vi "LOX Crossover Template.vi"(6 "Array Size":i32=9, 8 "Index 2":i32=5, 9 "Index 1":i32=3, 10 "Schedule 2":u16[](array[numeric])=[3, 7, 8, 1, 4, 9, 2, 5, 6], 11 "Schedule 1":u16[](array[numeric])=[1, 3, 2, 6, 4, 5, 9, 7, 8]) -> (3 "Child":u16[](array[numeric]))   [LabVIEW 2013, in "GA.lvclass"]
uses:
  GA.lvclass
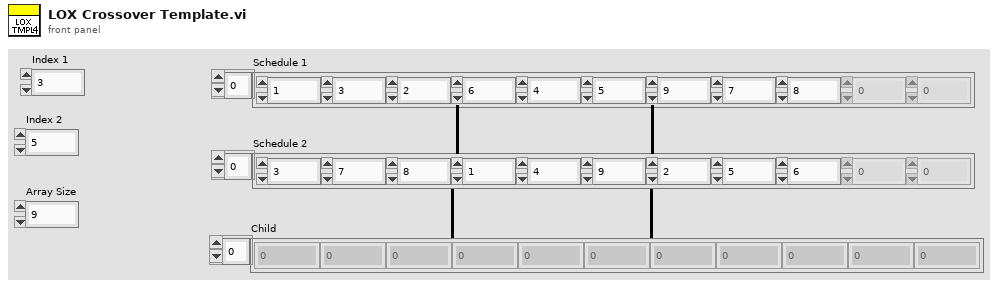
[diagram p1: front panel]
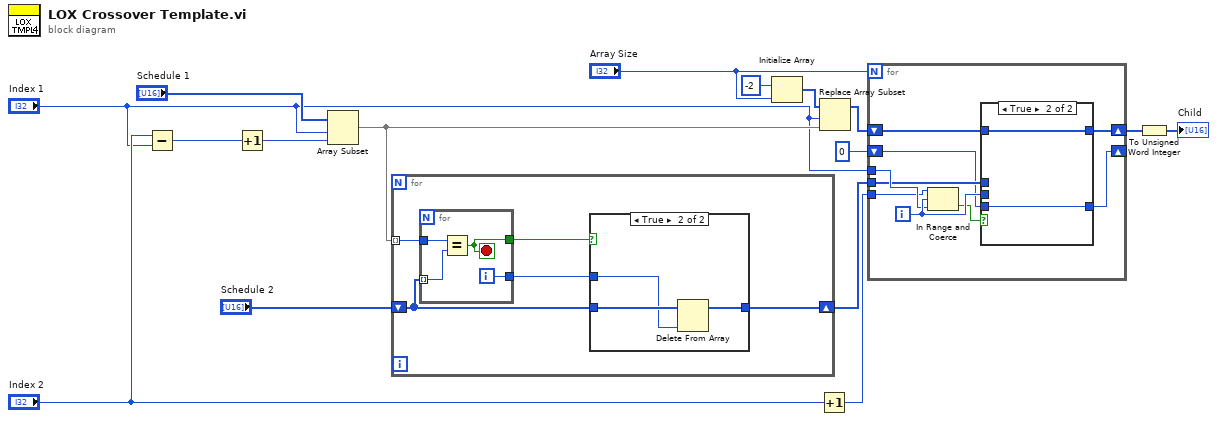
[diagram p0: block diagram]
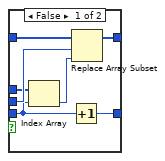
[diagram p2: hidden frame]
diagram:
  n1 = Subtract(x="Index 2", y="Index 1") -> (x-y=w14:i32)
  n2 = Increment(x=w14) -> (x+1=w13:i32)
  n3 = Array Subset(array="Schedule 1", index="Index 1", length=w13) -> (w10:u16[])
  n4 = for {
    shift-right: [w17] -> w7
    shift-left: "Schedule 2" -> [w19]
    tunnel: w10 -> [w21] mode=indexing
    n5 = for {
      tunnel: w19 -> [w28] mode=indexing
      tunnel: w21 -> [w29]
      tunnel: [w27] -> w20
      tunnel: [w26] -> w18
      i -> [w26]
      stop <- w27 stop-if-true
      n6 = Equal?(x=w29, y=w28) -> (x = y?=w27:bool)
    }
    n7 = case shown="True" w20 {
      tunnel: w19 -> [w22 w25]
      tunnel: w18 -> [_ w24]
      tunnel: [w22 w23] -> w17
      frame False {
      }
      frame True {
        n8 = Delete From Array(array=w25, index=w24) -> (array with subset deleted=w23:u16[])  [unwired: 1 in, 1 out]
      }
    }
  }
  n9 = Initialize Array(i16 -2 ("element"), "Array Size") -> (w11:i16[])
  n10 = Increment(x="Index 2") -> (x+1=w8:i32)
  n11 = Replace Array Subset(array=w11, new element=w10, index="Index 1") -> (w9:i16[])
  n12 = for {
    N: "Array Size" -> [_]
    tunnel: w8 -> [w33]
    tunnel: w7 -> [w32]
    shift-right: [w37] -> w6
    shift-left: w9 -> [w38]
    tunnel: "Index 1" -> [w34]
    shift-right: [w30] -> _
    shift-left: 0 -> [w31]
    i -> [w36]
    n13 = In Range and Coerce(upper limit=w33, x=w36, lower limit=w34) -> (In Range?=w35:bool)  [unwired: 1 out]
    n14 = case shown="True" w35 {
      tunnel: w38 -> [w45 w47]
      tunnel: [w44 w47] -> w37
      tunnel: w36 -> [w43 _]
      tunnel: w32 -> [w42 _]
      tunnel: w31 -> [w40 w46]
      tunnel: [w39 w46] -> w30
      frame False {
        n15 = Index Array(array=w42, index=w40) -> (element=w41:u16)
        n16 = Increment(x=w40) -> (x+1=w39:i32)
        n17 = Replace Array Subset(array=w45, new element=w41, index=w43) -> (w44:i16[])
      }
      frame True {
      }
    }
  }
  n18 = To Unsigned Word Integer(number=w6) -> (unsigned 16bit integer=→"Child":u16[])
